vi "Create_Additional_NIPaths.vi"(8 "error in (no error)":errorcluster, 11 "Installer in":refnum<class "Installer.lvclass">) -> (0 "error out":errorcluster, 3 "Installer out":refnum<class "Installer.lvclass">)   [LabVIEW 2020, in "Installer.lvclass"]
uses:
  <vilib>/AppBuilder/IB_Classes/Installer/Installer.lvclass
  <vilib>/AppBuilder/IB_Classes/Installer/Installer.lvclass/Installer.ctl
  <vilib>/AppBuilder/IB_Classes/Dest_NI_NIPath/Dest_NI_NIPath.lvclass
  <vilib>/AppBuilder/IB_Classes/Destination/IB_Destination.lvclass
  e:/builds/penguin/labview/branches/2020/dev/dist/vi.lib/AppBuilder/IB_Classes/Destination/niLabel/niLabel.lvclass
  e:/builds/penguin/labview/branches/2020/dev/dist/vi.lib/AppBuilder/IB_Classes/Destination/IB_Destination.lvclass
  e:/builds/penguin/labview/branches/2020/dev/dist/vi.lib/AppBuilder/IB_Classes/Dest_NI_NIPath/Dest_NI_NIPath.lvclass
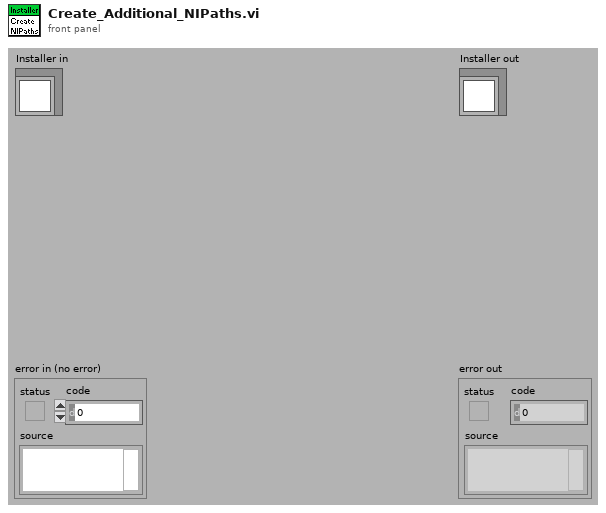
[diagram p1: front panel]
types:
  T1 = typedef "IB_Destination.ctl" = cluster{"name":string, "unlock":bool, "parentTag":string, "destTag":string, "eng_installPath":string}
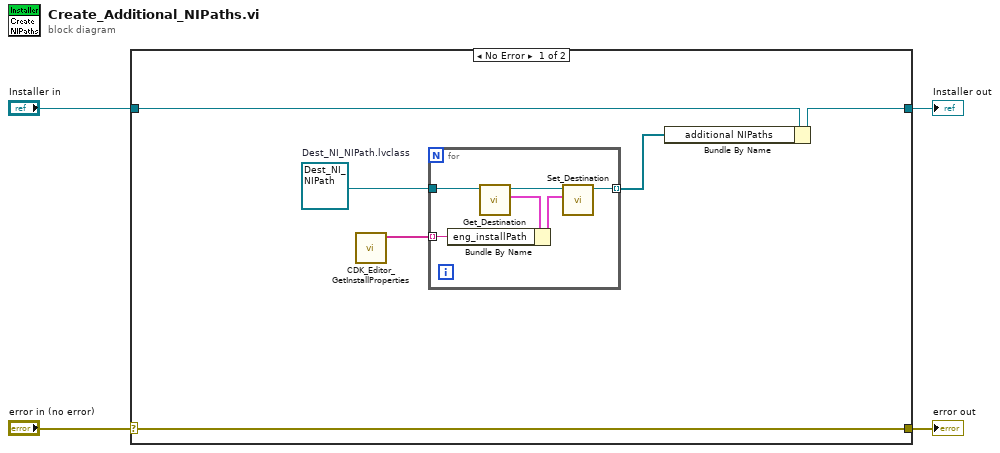
[diagram p0: block diagram]
diagram:
  n1 = case shown="No Error" "error in (no error)" {
    selector: "error in (no error)" -> [w10 w18]
    tunnel: [w10 w18] -> w3
    tunnel: [w7 w17] -> w1
    tunnel: "Installer in" -> [w8 w17]
    frame No Error {
      w9 = refnum<class "Dest_NI_NIPath.lvclass"> refnum  # Dest_NI_NIPath.lvclass
      n2 = call <resource>:"CDK_Editor_GetInstallProperties.vi"() -> ("install properties"=w5:string[])  [unwired: 11 in]
      n3 = for {
        tunnel: w9 -> [w13]
        tunnel: [w12] -> w6 mode=indexing
        tunnel: w5 -> [w11] mode=indexing
        n4 = call <vilib>:"Get_Destination.vi"("IB_Destination in"=w13) -> ("data"=w15:T1, "IB_Destination out"=w16:refnum<class "Dest_NI_NIPath.lvclass">)  [unwired: 1 in, 8 out]
        n5 = Bundle By Name(cluster=w15, "eng_installPath"=w11) -> (w14:T1)
        n6 = call <vilib>:"Set_Destination.vi"("data"=w14, "IB_Destination in"=w16) -> ("IB_Destination out"=w12:refnum<class "Dest_NI_NIPath.lvclass">)  [unwired: 1 in, 8 out]
      }
      n7 = Bundle By Name(cluster=w8, "additional NIPaths"=w6) -> (w7:refnum<class "Installer.lvclass">)
    }
    frame Error {
    }
  }
  "error out" <- w3
  "Installer out" <- w1
